vi "Main_lidar2grid-map.vi"() -> ()   [LabVIEW 2019]
uses:
  <vilib>/Analysis/Matrix/Datatypes/RealMatrix.ctl
  Ctrl/cmd_common.ctl
  <vilib>/Utility/file.llb/Read Delimited Spreadsheet (DBL).vi
  <vilib>/Analysis/Matrix/NI_Matrix.lvlib
panel:
  in  "tab":enum32{"페이지 1", "페이지 2"}(tab)
  in  "xy_resolution":dbl=0.02
  in  "EXTEND_AREA":dbl=1.0
  out "i":i32
  out "Raw map":cluster{"X":dbl, "Y":dbl}[](graph)
  out "Occupacy Grid Map":dbl[][](graph)
  out "occupancy map":T1
  # "Lidar to Gridmap"
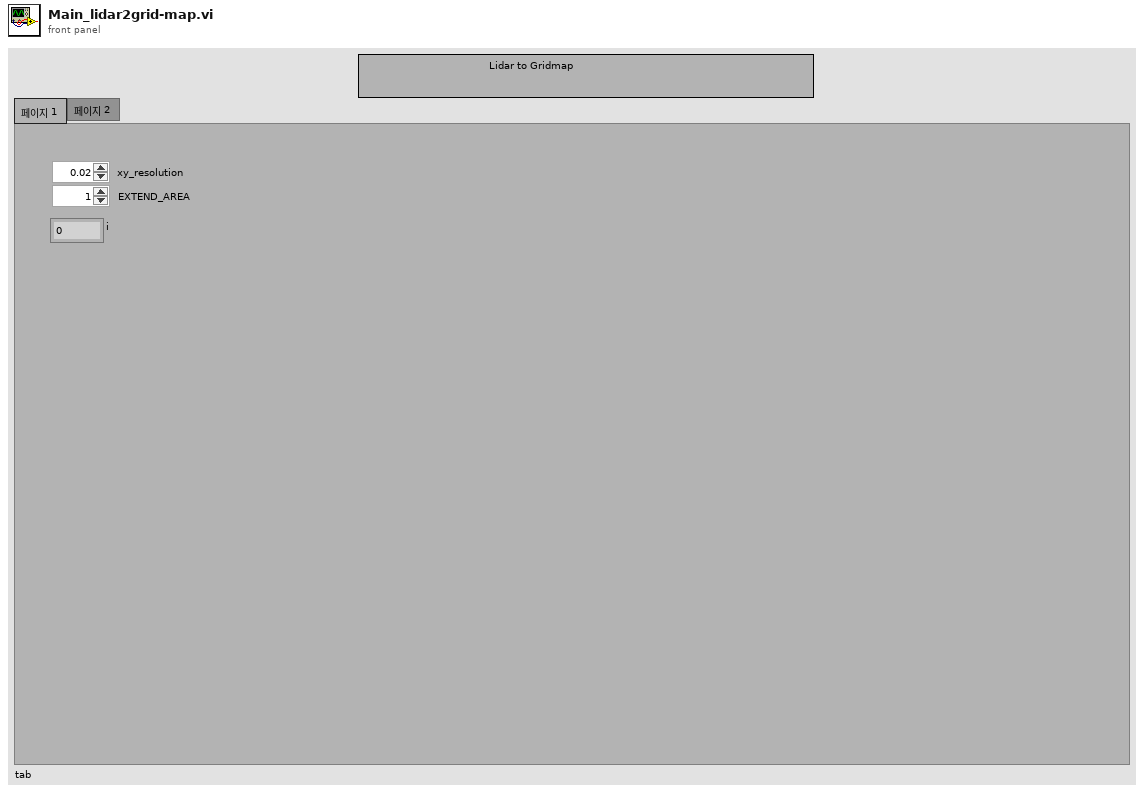
[diagram p1: front panel]
types:
  T1 = typedef "NI_Matrix.lvlib/RealMatrix.ctl" = dbl[][]
  T2 = typedef "cmd_common.ctl" = enum16{"read", "write"}
  T3 = cluster{"xy_resolution":dbl, "EXTEND_AREA":dbl, "MAX_RANGE":dbl, "NP":u32, "NTh":u32, "Q":T1, "R":T1, "Q_sim":T1, "R_sim":T1, "rf_id":cluster{"x":dbl, "y":dbl}[]}
  T4 = cluster{"ox":dbl[], "oy":dbl[], "occupancy map":T1, "x_true":T1, "u":T1, "z":T1, "PEst":T1, "min x":dbl, "min y":dbl, "max x":dbl, "max y":dbl, "yw":i32, "xw":i32, "center x":i32, "center y":i32}
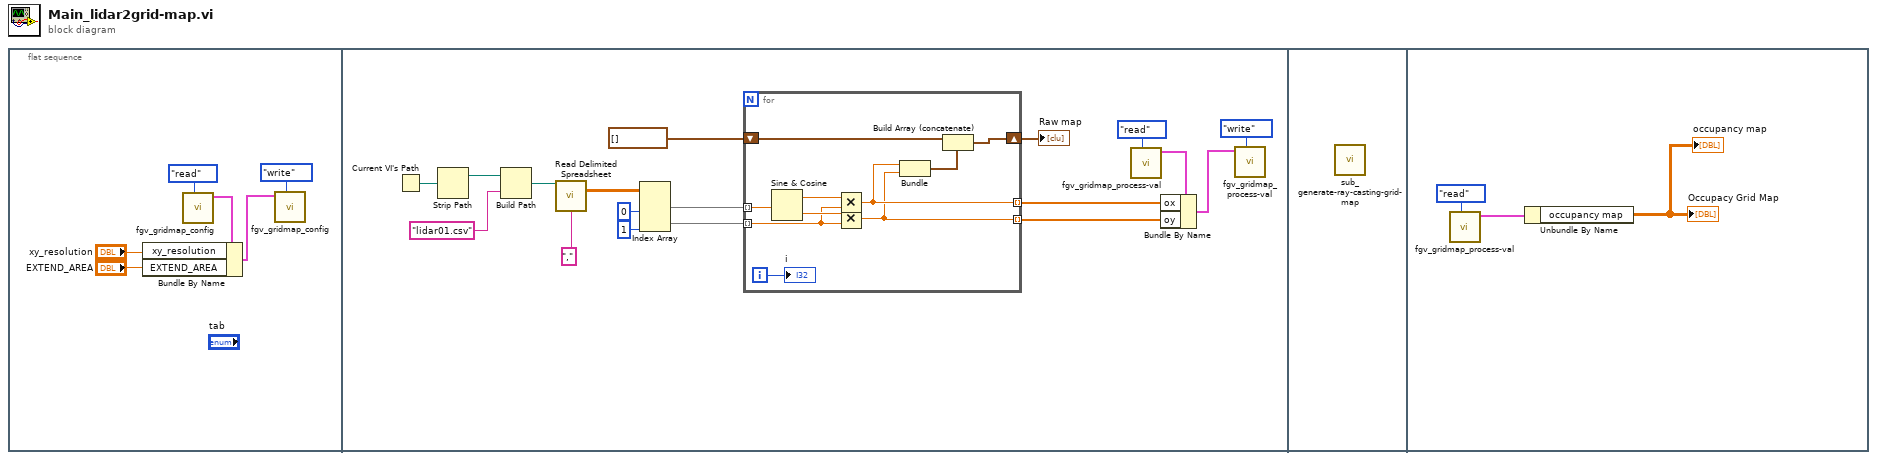
[diagram p0: block diagram]
diagram:
  n1 = flat-sequence {
    frame #0 {
      n2 = call "fgv_gridmap_config.vi"("cmd"=cmd_common."read") -> ("pf-val out"=w4:T3)  [unwired: 10 in]
      n3 = Bundle By Name(cluster=w4, "xy_resolution"="xy_resolution", "EXTEND_AREA"="EXTEND_AREA") -> (w2:T3)
      n4 = call "fgv_gridmap_config.vi"("cmd"=cmd_common."write", "pf-val"=w2) -> ()  [unwired: 9 in, 1 out]
    }
    frame #1 {
      n5 = Current VI's Path() -> (path=w16:path)
      n6 = Strip Path(path=w16) -> (stripped path=w15:path)  [unwired: 1 out]
      n7 = Build Path(base path=w15, name or relative path="lidar01.csv" ("이름 또는 상대 경로")) -> (appended path=w13:path)
      n8 = call-poly <vilib>:"Read Delimited Spreadsheet.vi"("file path (dialog if empty)"=w13, "delimiter (\\t)"="," ("delimiter (\\t)")) -> ("all rows"=w23:dbl[][])  [unwired: 8 in, 5 out]
      n9 = Index Array(array=w23, index (col) #1=0 ("비활성화된 인덱스 (열)"), index (col) #2=1 ("인덱스 (열)")) -> (element #1=w20:dbl[], element #2=w18:dbl[])  [unwired: 2 in]
      n10 = for {
        tunnel: w20 -> [w34] mode=indexing
        shift-right: [w28] -> w17
        shift-left: cluster{"x":dbl, "y":dbl}[] [] -> [w33]
        tunnel: w18 -> [w30] mode=indexing
        tunnel: [w26] -> w8 mode=indexing
        tunnel: [w25] -> w7 mode=indexing
        i -> [w27]
        n11 = Sine & Cosine(0:w34) -> (1:w32:dbl, 2:w31:dbl)
        n12 = Multiply(x=w32, y=w30) -> (x*y=w26:dbl)
        n13 = Multiply(x=w31, y=w30) -> (x*y=w25:dbl)
        n14 = Bundle(w26, w25) -> (w29:cluster{dbl, dbl})  [unwired: 1 in]
        n15 = Build Array (concatenate)(w33, w29) -> (w28:cluster{"x":dbl, "y":dbl}[])
        "i" <- w27
      }
      "Raw map" <- w17
      n16 = call "fgv_gridmap_process-val.vi"("cmd"=cmd_common."read") -> ("p-val  2"=w10:T4)  [unwired: 10 in]
      n17 = Bundle By Name(cluster=w10, "ox"=w8, "oy"=w7) -> (w9:T4)
      n18 = call "fgv_gridmap_process-val.vi"("cmd"=cmd_common."write", "p-val"=w9) -> ()  [unwired: 9 in, 1 out]
    }
    frame #2 {
      n19 = call "sub_generate-ray-casting-grid-map.vi"() -> ()  [unwired: 12 in]
    }
    frame #3 {
      n20 = call "fgv_gridmap_process-val.vi"("cmd"=cmd_common."read") -> ("p-val  2"=w36:T4)  [unwired: 10 in]
      n21 = Unbundle By Name(w36) -> ("occupancy map"=→"Occupacy Grid Map" →"occupancy map":T1)
    }
  }
